vi "test_all_riccati.vi"(8 "error in (no error)":errorcluster) -> (0 "error out":errorcluster, 3 "All Tests Passed":bool)   [LabVIEW 2019]
panel:
  out "Test 5":bool
  out "Test 4":bool
  out "Test 3":bool
  out "Test 2":bool
  out "Test 1":bool
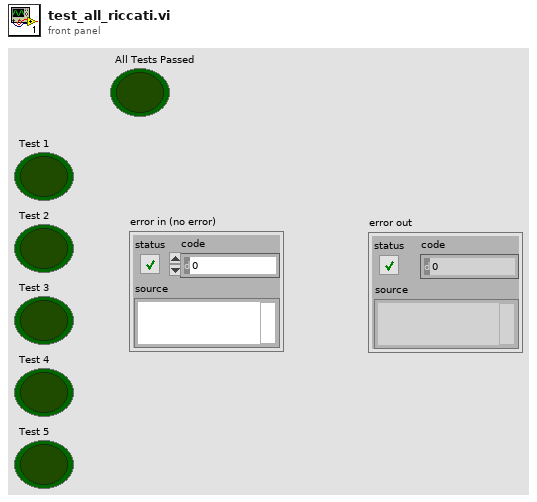
[diagram p1: front panel]
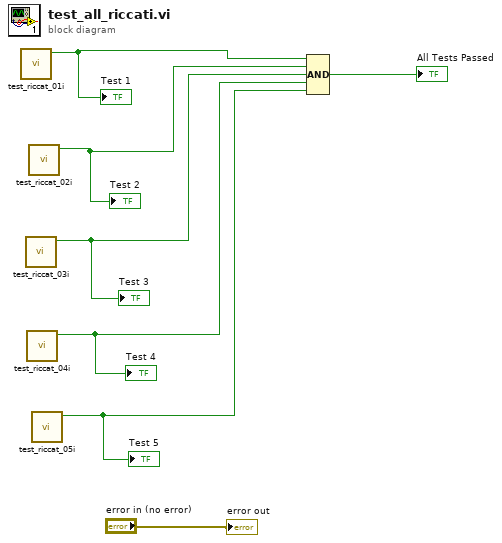
[diagram p0: block diagram]
diagram:
  n1 = call "test_riccat_01i.vi"() -> ("All Tests Passed"=w6:bool)  [unwired: 11 in]
  "Test 1" <- w6
  n2 = call "test_riccat_03i.vi"() -> ("All Tests Passed"=w4:bool)  [unwired: 11 in]
  "Test 3" <- w4
  n3 = call "test_riccat_04i.vi"() -> ("All Tests Passed"=w3:bool)  [unwired: 11 in]
  "Test 4" <- w3
  n4 = call "test_riccat_02i.vi"() -> ("All Tests Passed"=w5:bool)  [unwired: 11 in]
  "Test 2" <- w5
  n5 = call "test_riccat_05i.vi"() -> ("All Tests Passed"=w2:bool)  [unwired: 11 in]
  "Test 5" <- w2
  n6 = Compound Arithmetic op=AND(w6, w5, w4, w3, w2) -> (→"All Tests Passed":bool)
  "error out" <- "error in (no error)"
